vi "Alltesta Connect.vi"(8 "error in (no error)":errorcluster, 11 "VISA resource name":refnum<visa-resource-name>) -> (0 "error out":errorcluster, 3 "VISA resource name out":refnum<visa-resource-name>)   [LabVIEW 2023, in "Alltesta Autosampler.lvlib"]
uses:
  Alltesta Autosampler.lvlib
  <vilib>/Instr/_visa.llb/VISA Flush IO Buffer Mask.ctl
  <vilib>/Instr/_visa.llb/VISA Configure Serial Port (Instr).vi
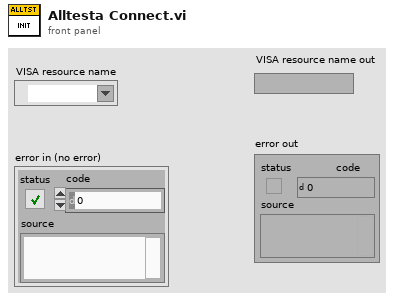
[diagram p1: front panel]
types:
  T1 = typedef "VISA Flush IO Buffer Mask.ctl" = u16
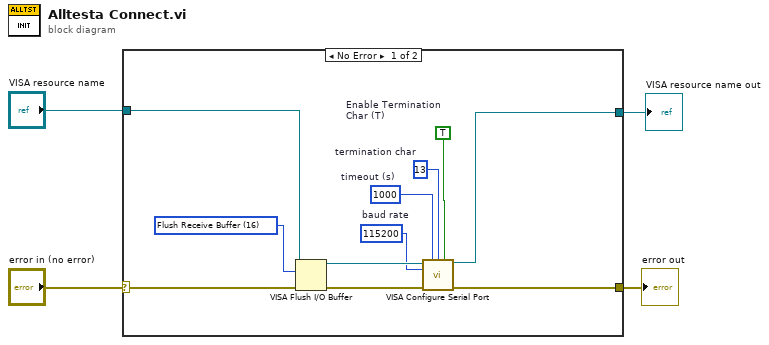
[diagram p0: block diagram]
diagram:
  n1 = case shown="No Error" "error in (no error)" {
    selector: "error in (no error)" -> [w6 w17]
    tunnel: [w9 w17] -> w4
    tunnel: "VISA resource name" -> [w8 w16]
    tunnel: [w7 w16] -> w2
    frame No Error {
      w5 = u32 1000  # timeout (s)
      w10 = u8 13  # termination char
      w11 = TRUE  # Enable Termination Char (T)
      w12 = u32 115200  # baud rate
      w15 = T1 16 items=["Flush Receive Buffer"=16, "Write Transmit Buffer to Device"=32, "Flush Receive Buffer (No I/O)"=64, "Flush Transmit Buffer"=128] ("Mask")
      n2 = VISA Flush I/O Buffer(VISA resource name=w8, mask (16)=w15, error in (no error)=w6) -> (VISA resource name out=w13:refnum<visa-resource-name>, error out=w14:errorcluster)
      n3 = call-poly "VISA Configure Serial Port"("VISA resource name"=w13, "timeout (10sec)"=w5, "termination char\n(0xA = '\\n' = LF)"=w10, "Enable Termination\nChar (T)"=w11, "baud rate (9600)"=w12, "error in (no error)"=w14) -> ("VISA resource name out"=w7:refnum<visa-resource-name>, "error out"=w9:errorcluster)  [unwired: 8 in]
    }
    frame Error {
    }
  }
  "error out" <- w4
  "VISA resource name out" <- w2
